vi "Configuration Process.vi"(8 "error in (no error)":errorcluster, 11 "View Model":T1) -> (0 "error out":errorcluster)   [LabVIEW 2017]
doc: "The Configuration process used by the Controller\nto read and update DB Records\n[Covers: CD4]"
uses:
  View Model/Controls/View Model.ctl
  View Model/Controls/Shared Model.ctl
  Error/Controls/Error Model.ctl
  Error/Controls/Error Event.ctl
  Error/Controls/Error Type.ctl
  Controls/Config DB Model.ctl
  Controls/Config DB Command.ctl
  Controls/Config DB Record.ctl
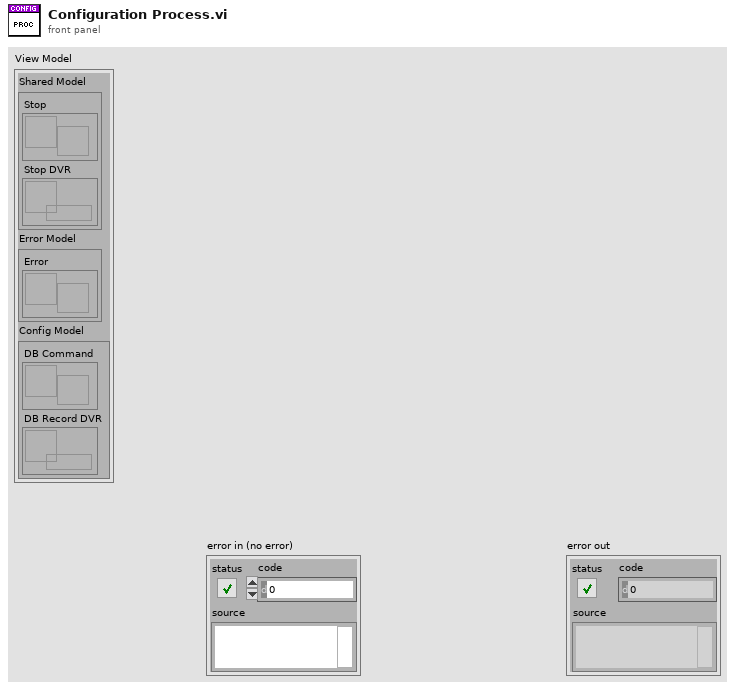
[diagram p1: front panel]
types:
  T1 = typedef "View Model.ctl" = cluster{"Shared Model":T2, "Error Model":T3, "Config Model":T4}
  T2 = typedef "Shared Model.ctl" = cluster{"Stop":refnum<user-event>, "Stop DVR":refnum<data-value>}
  T3 = typedef "Error Model.ctl" = cluster{"Error":refnum<user-event>}
  T4 = typedef "Config DB Model.ctl" = cluster{"DB Command":refnum<user-event>, "DB Record DVR":refnum<data-value>}
  T5 = typedef "Config DB Command.ctl" = enum16{"Read", "Update"}
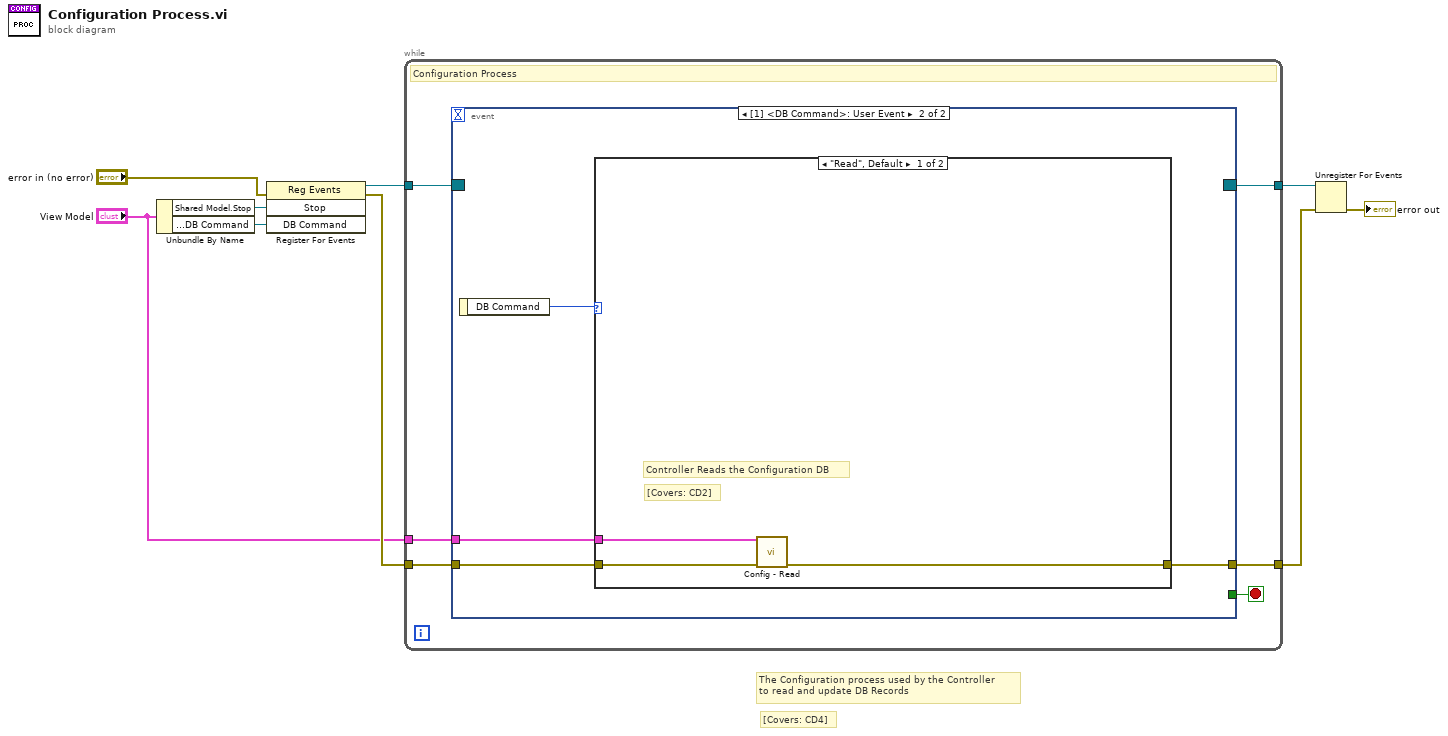
[diagram p0: block diagram]
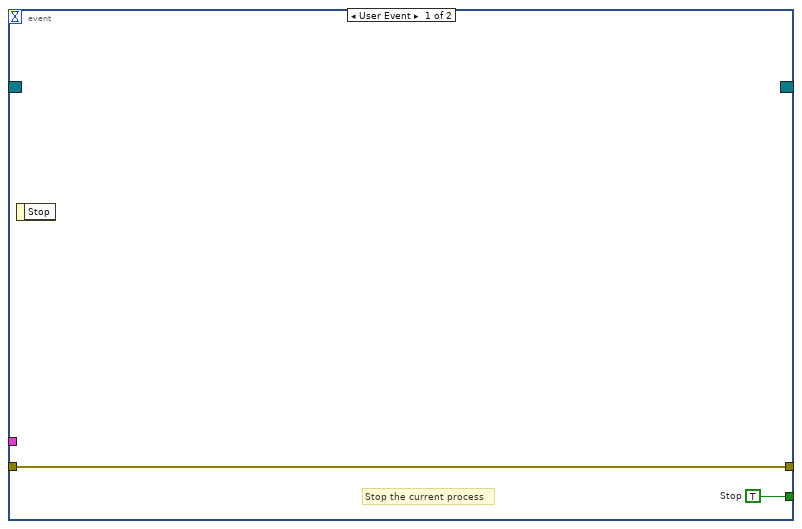
[diagram p2: hidden frame]
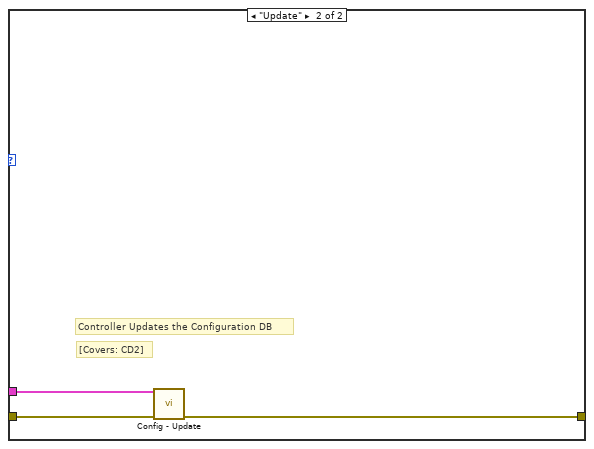
[diagram p3: hidden frame]
diagram:
  # "[Covers: CD4]"
  # "The Configuration process used by the Controller\nto read and update DB Records"
  n1 = Unbundle By Name("View Model") -> ("Shared Model.Stop"=w9:refnum<user-event>, "Config Model.DB Command"=w1:refnum<user-event>)
  n2 = register-events(error in="error in (no error)", w9, w1) -> (reference out=w8:refnum<event-registration>, error out=w5:errorcluster)  [unwired: 1 in]
  n3 = while {
    tunnel: w8 -> [w15]
    tunnel: [w14] -> w7
    tunnel: w5 -> [w13]
    tunnel: "View Model" -> [w12]
    tunnel: [w11] -> w3
    stop <- w10 stop-if-true
    # "Configuration Process"
    n4 = event shown="[1] <DB Command>: User Event" {
      selector: w15 -> [_ _]
      dyn-events: [_ _] -> w14
      timeout: _ -> [_ _]
      tunnel: w13 -> [w17 w19]
      tunnel: w12 -> [_ w20]
      tunnel: [w17 w18] -> w11
      tunnel: [w16 _] -> w10
      event User Event {
        w16 = TRUE  # Stop
        # "Stop the current process"
        n5 = event-data() -> ()  [unwired: 1 in, 1 out]
      }
      event User Event {
        n6 = event-data() -> ("DB Command"=w21:T5)  [unwired: 1 in]
        n7 = case shown="\"Read\", Default" w21 {
          tunnel: w20 -> [w24 w26]
          tunnel: w19 -> [w23 w27]
          tunnel: [w22 w25] -> w18
          frame "Read", Default {
            # "[Covers: CD2]"
            # "Controller Reads the Configuration DB"
            n8 = call "Config - Read.vi"("error in (no error)"=w23, "View Model"=w24) -> ("error out"=w22:errorcluster)  [unwired: 8 in, 1 out]
          }
          frame "Update" {
            # "[Covers: CD2]"
            # "Controller Updates the Configuration DB"
            n9 = call "Config - Update.vi"("error in (no error)"=w27, "View Model"=w26) -> ("error out"=w25:errorcluster)  [unwired: 8 in, 1 out]
          }
        }
      }
    }
  }
  n10 = Unregister For Events(event registration refnum=w7, error in=w3) -> (error out=→"error out":errorcluster)
